vi "Configure Session.vi"(8 "error in":errorcluster, 11 "Plugin in":refnum<class "Spectrogram.lvclass">) -> (0 "error out":errorcluster, 3 "Plugin out":refnum<class "Spectrogram.lvclass">)   [LabVIEW 2023, in "Spectrogram.lvlib" / "Spectrogram.lvclass"]
uses:
  Spectrogram.lvclass
  C:/Program Files/National Instruments/LabVIEW 2023/vi.lib/FlexLogger/SDK/PluginSDK.lvlibp/PEFClasses/SDK/Plugin/Plugin.lvclass
  Spectrogram Data.ctl
  Spectrogram.lvclass/Spectrogram.ctl
  Spectrogram Global.vi
  <vilib>/FlexLogger/SDK/PluginSDK.lvlibp/PEFClasses/SDK/Plugin/ParameterAccess/Read Enum.vi
  <vilib>/FlexLogger/SDK/PluginSDK.lvlibp/PEFClasses/SDK/Plugin/ParameterAccess/Read I32.vi
  <vilib>/FlexLogger/SDK/PluginSDK.lvlibp/PEFClasses/SDK/Plugin/Plugin.lvclass
  C:/Program Files/National Instruments/LabVIEW 2023/vi.lib/FlexLogger/SDK/PluginSDK.lvlibp/PEFClasses/SDK/Processing Element/Processing Element.lvclass
  C:/Users/Localization Tester/Documents/LabVIEW Projects/FlexLogger IO Plug-ins/Spectrogram/Spectrogram.lvclass
  <vilib>/Utility/LVLibp/NI_PackedLibraryUtility.lvlib
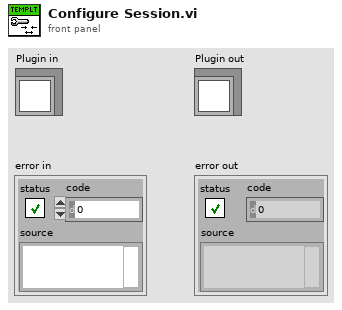
[diagram p1: front panel]
types:
  T1 = typedef "Spectrogram.lvlib/Spectrogram.lvclass/Spectrogram Data.ctl" = cluster{"First Time":bool, "Show Spectrogram Window":bool, "Show Spectrogram Window Button Clicked":bool, "Extension":u16, "Time steps":i32, "Frequency bins":i32, "Type":i32, "Length":i32, "Color Table":u16, "Spectrogram VI Ref":refnum<vi>}
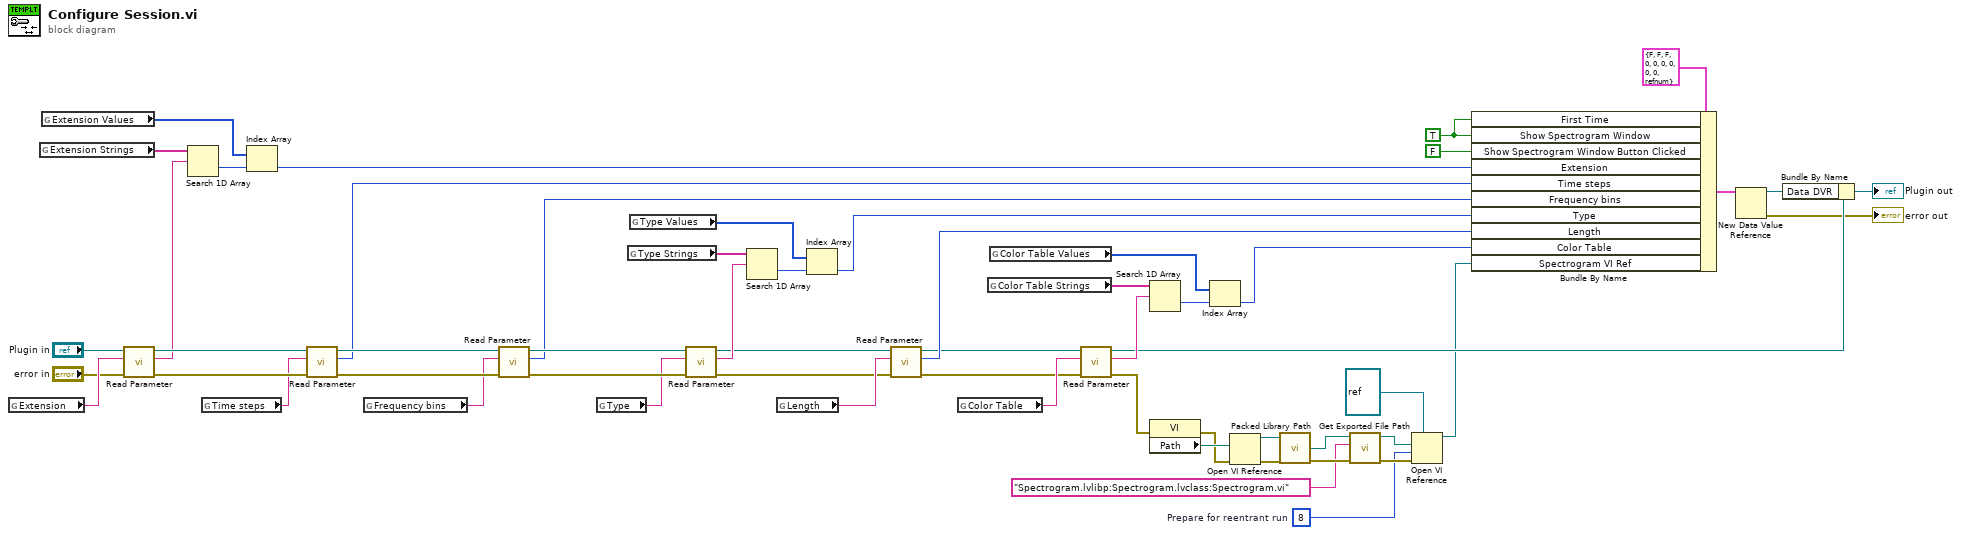
[diagram p0: block diagram]
diagram:
  w6 = 8  # Prepare for reentrant run
  w16 = TRUE ("Show Spectrogram Window")
  n1 = global read "Spectrogram Global.vi" "Extension"() -> (w51:string)
  n2 = global read "Spectrogram Global.vi" "Extension Strings"() -> (w50:string[])
  n3 = global read "Spectrogram Global.vi" "Extension Values"() -> (w48:u16[])
  n4 = call-poly <vilib>:"Read Parameter.vi"("error in (no error)"="error in", "Name"=w51, "Plugin in"="Plugin in") -> ("error out"=w56:errorcluster, "Value"=w49:string, "Plugin out"=w57:refnum<class "Spectrogram.lvclass">)  [unwired: 4 in, 2 out]
  n5 = Search 1D Array(1D array=w50, element=w49) -> (index of element=w47:i32)  [unwired: 1 in]
  n6 = global read "Spectrogram Global.vi" "Time steps"() -> (w46:string)
  n7 = Index Array(array=w48, index=w47) -> (element=w39:u16)
  n8 = call-poly <vilib>:"Read Parameter.vi"("error in (no error)"=w56, "Name"=w46, "Plugin in"=w57) -> ("error out"=w54:errorcluster, "Value"=w35:i32, "Plugin out"=w55:refnum<class "Spectrogram.lvclass">)  [unwired: 5 in, 1 out]
  n9 = global read "Spectrogram Global.vi" "Frequency bins"() -> (w45:string)
  n10 = call-poly <vilib>:"Read Parameter.vi"("error in (no error)"=w54, "Name"=w45, "Plugin in"=w55) -> ("error out"=w52:errorcluster, "Value"=w34:i32, "Plugin out"=w53:refnum<class "Spectrogram.lvclass">)  [unwired: 5 in, 1 out]
  n11 = global read "Spectrogram Global.vi" "Type"() -> (w40:string)
  n12 = global read "Spectrogram Global.vi" "Type Strings"() -> (w44:string[])
  n13 = global read "Spectrogram Global.vi" "Type Values"() -> (w43:i32[])
  n14 = call-poly <vilib>:"Read Parameter.vi"("error in (no error)"=w52, "Name"=w40, "Plugin in"=w53) -> ("error out"=w33:errorcluster, "Value"=w41:string, "Plugin out"=w36:refnum<class "Spectrogram.lvclass">)  [unwired: 4 in, 2 out]
  n15 = Search 1D Array(1D array=w44, element=w41) -> (index of element=w42:i32)  [unwired: 1 in]
  n16 = global read "Spectrogram Global.vi" "Length"() -> (w37:string)
  n17 = Index Array(array=w43, index=w42) -> (element=w38:i32)
  n18 = call-poly <vilib>:"Read Parameter.vi"("error in (no error)"=w33, "Name"=w37, "Plugin in"=w36) -> ("error out"=w25:errorcluster, "Value"=w32:i32, "Plugin out"=w26:refnum<class "Spectrogram.lvclass">)  [unwired: 5 in, 1 out]
  n19 = global read "Spectrogram Global.vi" "Color Table"() -> (w27:string)
  n20 = global read "Spectrogram Global.vi" "Color Table Strings"() -> (w31:string[])
  n21 = global read "Spectrogram Global.vi" "Color Table Values"() -> (w30:u16[])
  n22 = call-poly <vilib>:"Read Parameter.vi"("error in (no error)"=w25, "Name"=w27, "Plugin in"=w26) -> ("error out"=w4:errorcluster, "Value"=w28:string, "Plugin out"=w20:refnum<class "Spectrogram.lvclass">)  [unwired: 4 in, 2 out]
  n23 = Search 1D Array(1D array=w31, element=w28) -> (index of element=w29:i32)  [unwired: 1 in]
  n24 = property class="VI"(error in=w4) -> (error out=w9:errorcluster, "Path"=w15:path)  [unwired: 1 in, 1 out]
  n25 = Index Array(array=w30, index=w29) -> (element=w24:u16)
  n26 = Open VI Reference(vi path=w15, error in (no error)=w9) -> (vi reference=w14:refnum<vi>, error out=w13:errorcluster)  [unwired: 4 in]
  n27 = call <vilib>:"Packed Library Path.vi"("error in (no error)"=w13, "vi reference"=w14) -> ("error out"=w11:errorcluster, "packed library path"=w12:path)  [unwired: 1 in, 1 out]
  n28 = call <vilib>:"Get Exported File Path.vi"("error in (no error)"=w11, "qualified name"="Spectrogram.lvlibp:Spectrogram.lvclass:Spectrogram.vi", "packed library path"=w12) -> ("error out"=w7:errorcluster, "path"=w8:path)  [unwired: 7 in]
  n29 = Open VI Reference(type specifier VI Refnum (for type only)=refnum<vi> refnum, vi path=w8, options=w6, error in (no error)=w7) -> (vi reference=w3:refnum<vi>)  [unwired: 2 in, 1 out]
  n30 = Bundle By Name(cluster=T1 {"First Time"=FALSE, "Show Spectrogram Window"=FALSE, "Show Spectrogram Window Button Clicked"=FALSE, "Extension"=0, "Time steps"=0, "Frequency bins"=0, "Type"=0, "Length"=0, "Color Table"=0, "Spectrogram VI Ref"=refnum} ("Data"), "First Time"=w16, "Show Spectrogram Window"=w16, "Show Spectrogram Window Button Clicked"=FALSE ("Show Spectrogram Window"), "Extension"=w39, "Time steps"=w35, "Frequency bins"=w34, "Type"=w38, "Length"=w32, "Color Table"=w24, "Spectrogram VI Ref"=w3) -> (w22:T1)
  n31 = New Data Value Reference(data value=w22) -> (data value reference=w19:refnum<data-value>, error out=→"error out":errorcluster)  [unwired: 1 in]
  n32 = Bundle By Name(cluster=w20, "Data DVR"=w19) -> (→"Plugin out":refnum<class "Spectrogram.lvclass">)
